vi "res_Set Resistance.vi"(8 "error in (no error)":errorcluster, 9 "Resistance (0-65535 Ohms)":dbl min=0.0 max=65535.0 step=1.0, 10 "Channel (1-10)":i8=1 min=1 max=66 step=1 format="%.1f", 11 "instrument handle":refnum<visa-resource-name>) -> (0 "error out":errorcluster, 3 "instrument handle out":refnum<visa-resource-name>)   [LabVIEW 2014, in "Pickering 40-295.lvlib"]
doc: "VI shows how to control resistor values on a 40-290 board\nthe example is using a 16 bit dual resistor chain 0...32k Ohm.\n\nThis example VI uses the pi40 VISA driver. Resistance values in 0.5 ohm steps can be entered (0.0 to 32767.5) in the \"Enter Resistance Value\" field. The appropriate bit will be set and relays closed. \n\nAn OFF LED indicates an open relay and a resistance value included in the resistance chain. An ON LED indicates a closed switch, a resistance value shorted out and not included in the resistance chain."
uses:
  Pickering 40-295.lvlib
panel:
  out "Bit Pattern":u16 format="%016b"
  # "32768"
  # "16384"
  # "8192"
  # "4096"
  # "2048"
  # "1024"
  # "512"
  # "256"
  # "128"
  # "64"
  # "32"
  # "16"
  # "8"
  # "4"
  # "2"
  # "1"
  # "Max R   65535\nmin R 1 Ohm, 1 Ohm steps"
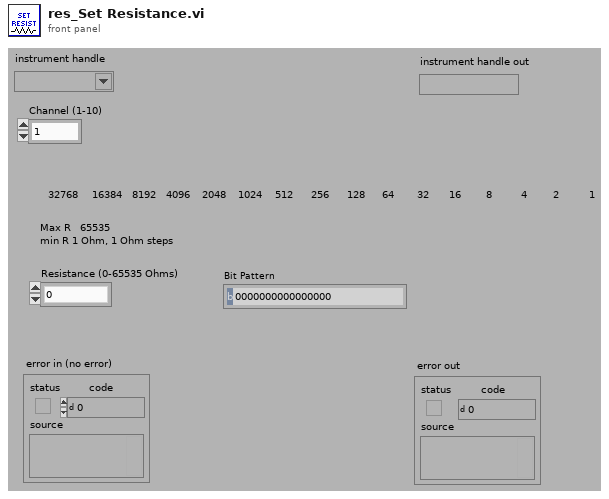
[diagram p1: front panel]
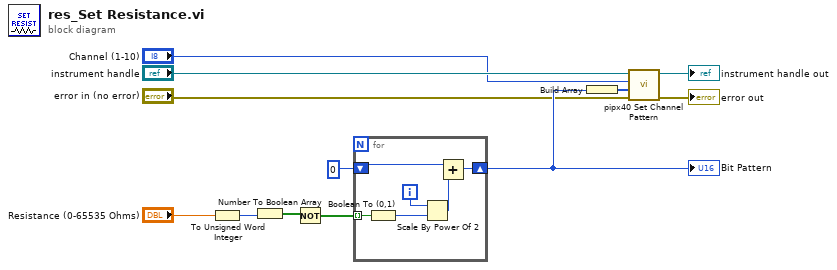
[diagram p0: block diagram]
diagram:
  n1 = To Unsigned Word Integer(number="Resistance (0-65535 Ohms)") -> (unsigned 16bit integer=w6:u16)
  n2 = Number To Boolean Array(number=w6) -> (Boolean array=w11:bool[])
  n3 = Not(x=w11) -> (.not. x?=w8:bool[])
  n4 = for {
    tunnel: w8 -> [w16] mode=indexing
    shift-right: [w13] -> w4
    shift-left: u16 0 -> [w14]
    i -> [w17]
    n5 = Boolean To (0,1)(Boolean=w16) -> (0, 1=w18:i16)
    n6 = Scale By Power Of 2(n=w17, x=w18) -> (x*2^n=w15:i16)
    n7 = Add(x=w14, y=w15) -> (x+y=w13:u16)
  }
  "Bit Pattern" <- w4
  n8 = Build Array(w4) -> (w3:u16[])
  n9 = call "pipx40 Set Channel Pattern.vi"("error in (no error)"="error in (no error)", "pattern"=w3, "subunit number"="Channel (1-10)", "instrument handle"="instrument handle") -> ("error out"=→"error out":errorcluster, "instrument handle out"=→"instrument handle out":refnum<visa-resource-name>)  [unwired: 6 out]
